vi "Stop Clone VIs (SubVI).vi"(8 "error in":errorcluster, 11 "Data Cluster in":T1={"VI References"=[], "Addresses"=[], "Pilot"=FALSE, "DO Data"=[], "Access Restricted?"=FALSE, "Pilot Control References"=[], "CoPilot Control References"=[], "cRIO Config"=[], "datalog Q"=refnum, "PS_P"={"AI"=[], "DI"=[], "DO"=[], "Serial"=[], "CPU"={"Total Load"=[], "Interrupt Load"=[], "Total Physical"=0.0, "Free Physical"=0.0, "Primary Disk Capacity"=0.0, "Primary Disk Free"=0.0}, "Stop"=FALSE, "DO Channel"=[]}, "PS_S"={"AI"=[], "DI"=[], "DO"=[], "Serial"=[], "CPU"={"Total Load"=[], "Interrupt Load"=[], "Total Physical"=0.0, "Free Physical"=0.0, "Primary Disk Capacity"=0.0, "Primary Disk Free"=0.0}, "Stop"=FALSE, "DO Channel"=[]}, "IDE_P"={"AI"=[], "DI"=[], "DO"=[], "Serial"=[], "CPU"={"Total Load"=[], "Interrupt Load"=[], "Total Physical"=0.0, "Free Physical"=0.0, "Primary Disk Capacity"=0.0, "Primary Disk Free"=0.0}, "Stop"=FALSE, "DO Channel"=[]}, "IDE_S"={"AI"=[], "DI"=[], "DO"=[], "Serial"=[], "CPU"={"Total Load"=[], "Interrupt Load"=[], "Total Physical"=0.0, "Free Physical"=0.0, "Primary Disk Capacity"=0.0, "Primary Disk Free"=0.0}, "Stop"=FALSE, "DO Channel"=[]}, "PDE_P"={"AI"=[], "DI"=[], "DO"=[], "Serial"=[], "CPU"={"Total Load"=[], "Interrupt Load"=[], "Total Physical"=0.0, "Free Physical"=0.0, "Primary Disk Capacity"=0.0, "Primary Disk Free"=0.0}, "Stop"=FALSE, "DO Channel"=[]}, "PDE_S"={"AI"=[], "DI"=[], "DO"=[], "Serial"=[], "CPU"={"Total Load"=[], "Interrupt Load"=[], "Total Physical"=0.0, "Free Physical"=0.0, "Primary Disk Capacity"=0.0, "Primary Disk Free"=0.0}, "Stop"=FALSE, "DO Channel"=[]}, "GUI References"={"Control Names"=[], "Control References"=[]}, "GUI Data"=[], "TCP - Serial"=[], "TCP-Serial Q"=refnum, "TCP Serial Ref"=[], "Data Sets"=[], "Last Data"=[], "Alarm Data"=[], "DI Data"=[], "Ack Data"=[], "Buzzer Data"=[], "Pilot DO"=[], "Co-Pilot DO"=[], "System Down?"=FALSE, "Log Data"=[], "Update Array"=[], "MCC Data Log"=[], "MCC Data Not"=refnum, "Thruster control"=[refnum, refnum, refnum, refnum, refnum, refnum, refnum, refnum, refnum], "waga notifier out"=refnum, "Wago  log"=[], "Thruster Cont"=[0.0, 0.0, 0.0, 0.0, 0.0, 0.0, 0.0, 0.0, 0.0], "Cam Cont"=[FALSE, FALSE, FALSE, FALSE, FALSE, TRUE], "PDE_P TH Cont"={"COM 10"=0.0, "COM 11"=0.0, "COM 12"=0.0, "COM 13"=0.0}, "PDE_S TH Cont"={"COM 10"=0.0, "COM 11"=0.0, "COM 12"=0.0, "COM 13"=0.0}} {"cRIO Config"."AI"."Interface Data"."Timing"."sample mode" items=["Finite Samples"=10178, "Continuous Samples"=10123, "Hardware Timed Single Point"=12522]; "cRIO Config"."Async"."Interface Data"."Data"."Minor Frame Count" min=5 max=8 step=1}) -> (0 "error out":errorcluster)   [LabVIEW 2021]
uses:
  Controls/Host - GUI Data Cluster.ctl
  Analog Output/Controls/AO JSON Data Cluster.ctl
  Analog Output/Controls/AO Interface Data Cluster.ctl
  Analog Output/Controls/AO Channel Configuration Cluster.ctl
  Analog Output/Controls/AO Timing Cluster.ctl
  Digital Output/Controls/DIO Configuration cluster.ctl
  Digital Output/Controls/DIO Interface Data.ctl
  Digital Output/SubVIs/Digital Dynamic Cluster.ctl
  Async JSON Cluster.ctl
  Async Interface Data Cluster.ctl
  Async Serial/Controls/Async Serial Configuration Cluster.ctl
  Async Serial/Controls/Async Frame Info Cluster.ctl
  Async Serial/Controls/Async Message Info Cluster.ctl
  Controls/Host Data Cluster.ctl
  Main Engine/Controls/Main Engine CPU Info.ctl
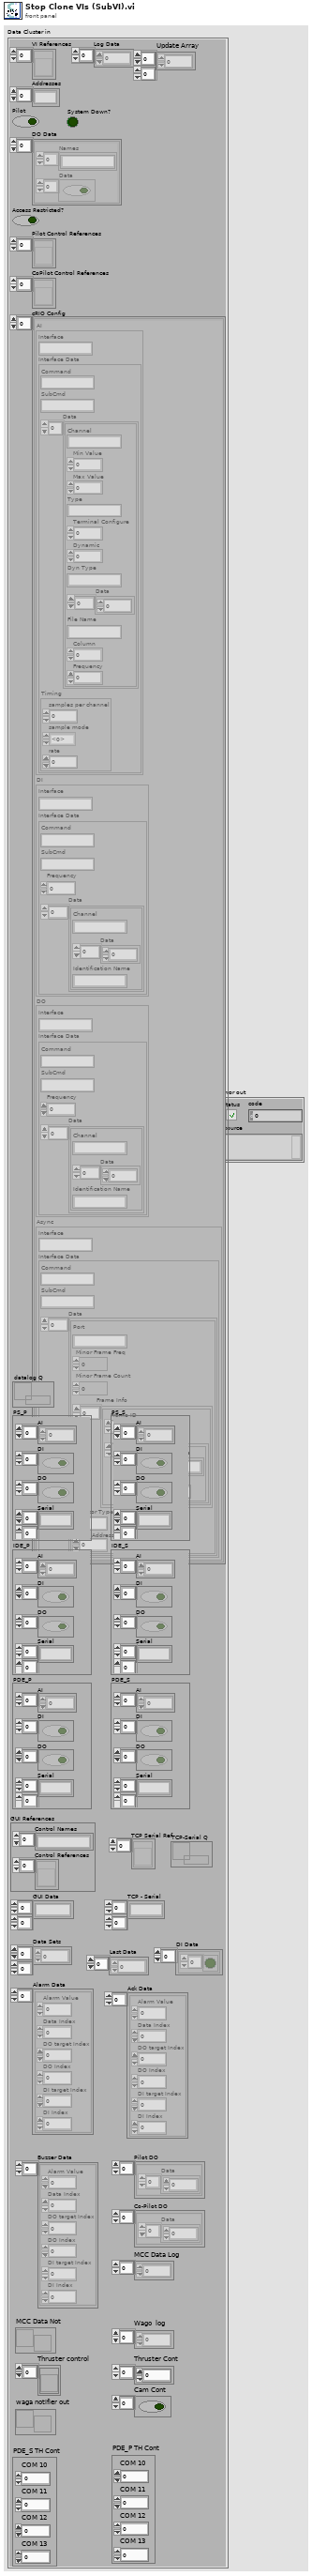
[diagram p1: front panel]
types:
  T1 = typedef "Host - GUI Data Cluster.ctl" = cluster{"VI References":refnum<vi>[], "Addresses":string[], "Pilot":bool, "DO Data":cluster{"Names":string[], "Data":bool[]}[], "Access Restricted?":bool, "Pilot Control References":refnum<vi>[], "CoPilot Control References":refnum<vi>[], "cRIO Config":cluster{"AI":T2, "DI":T6, "DO":T6, "Async":T9}[], "datalog Q":refnum<queue>, "PS_P":T14, "PS_S":T14, "IDE_P":T14, "IDE_S":T14, "PDE_P":T14, "PDE_S":T14, "GUI References":cluster{"Control Names":string[], "Control References":refnum<vi>[]}, "GUI Data":string[][], "TCP - Serial":string[][], "TCP-Serial Q":refnum<queue>, "TCP Serial Ref":refnum<vi>[], "Data Sets":dbl[][], "Last Data":dbl[], "Alarm Data":cluster{"Alarm Value":dbl, "Data Index":i32, "DO target Index":i32, "DO Index":i32, "DI target Index":i32, "DI Index":i32}[], "DI Data":cluster{bool[]}[], "Ack Data":cluster{"Alarm Value":dbl, "Data Index":i32, "DO target Index":i32, "DO Index":i32, "DI target Index":i32, "DI Index":i32}[], "Buzzer Data":cluster{"Alarm Value":dbl, "Data Index":i32, "DO target Index":i32, "DO Index":i32, "DI target Index":i32, "DI Index":i32}[], "Pilot DO":cluster{"Data":i32[]}[], "Co-Pilot DO":cluster{"Data":i32[]}[], "System Down?":bool, "Log Data":dbl[], "Update Array":i32[][], "MCC Data Log":dbl[], "MCC Data Not":refnum<notifier>, "Thruster control":refnum<vi>[], "waga notifier out":refnum<notifier>, "Wago  log":sgl[], "Thruster Cont":dbl[], "Cam Cont":bool[], "PDE_P TH Cont":cluster{"COM 10":dbl, "COM 11":dbl, "COM 12":dbl, "COM 13":dbl}, "PDE_S TH Cont":cluster{"COM 10":dbl, "COM 11":dbl, "COM 12":dbl, "COM 13":dbl}}
  T2 = typedef "AO JSON Data Cluster.ctl" = cluster{"Interface":string, "Interface Data":T3}
  T3 = typedef "AO Interface Data Cluster.ctl" = cluster{"Command":string, "SubCmd":string, "Data":T4[], "Timing":T5}
  T4 = typedef "AO Channel Configuration Cluster.ctl" = cluster{"Channel":string, "Min Value":dbl, "Max Value":dbl, "Type":string, "Terminal Configure":u16, "Dynamic":u8, "Dyn Type":string, "Data":dbl[], "File Name":string, "Column":i32, "Frequency":dbl}
  T5 = typedef "AO Timing Cluster.ctl" = cluster{"samples per channel":i32, "sample mode":i32, "rate":dbl}
  T6 = typedef "DIO Configuration cluster.ctl" = cluster{"Interface":string, "Interface Data":T7}
  T7 = typedef "DIO Interface Data.ctl" = cluster{"Command":string, "SubCmd":string, "Frequency":u16, "Data":T8[]}
  T8 = typedef "Digital Dynamic Cluster.ctl" = cluster{"Channel":string, "Data":u8[], "Identification Name":string}
  T9 = typedef "Async JSON Cluster.ctl" = cluster{"Interface":string, "Interface Data":T10}
  T10 = typedef "Async Interface Data Cluster.ctl" = cluster{"Command":string, "SubCmd":string, "Data":T11[]}
  T11 = typedef "Async Serial Configuration Cluster.ctl" = cluster{"Port":string, "Minor Frame Freq":u16, "Minor Frame Count":u16, "Frame Info":T12[], "Sensor Type":u16, "OIM Address":u16}
  T12 = typedef "Async Frame Info Cluster.ctl" = cluster{"Frame ID":u16, "Message Info":T13[]}
  T13 = typedef "Async Message Info Cluster.ctl" = cluster{"Message":u8[], "Message Name":string}
  T14 = typedef "Host Data Cluster.ctl" = cluster{"AI":dbl[], "DI":bool[], "DO":bool[], "Serial":string[][], "CPU":T15, "Stop":bool, "DO Channel":string[]}
  T15 = typedef "Main Engine CPU Info.ctl" = cluster{"Total Load":u32[], "Interrupt Load":u32[], "Total Physical":dbl, "Free Physical":dbl, "Primary Disk Capacity":dbl, "Primary Disk Free":dbl}
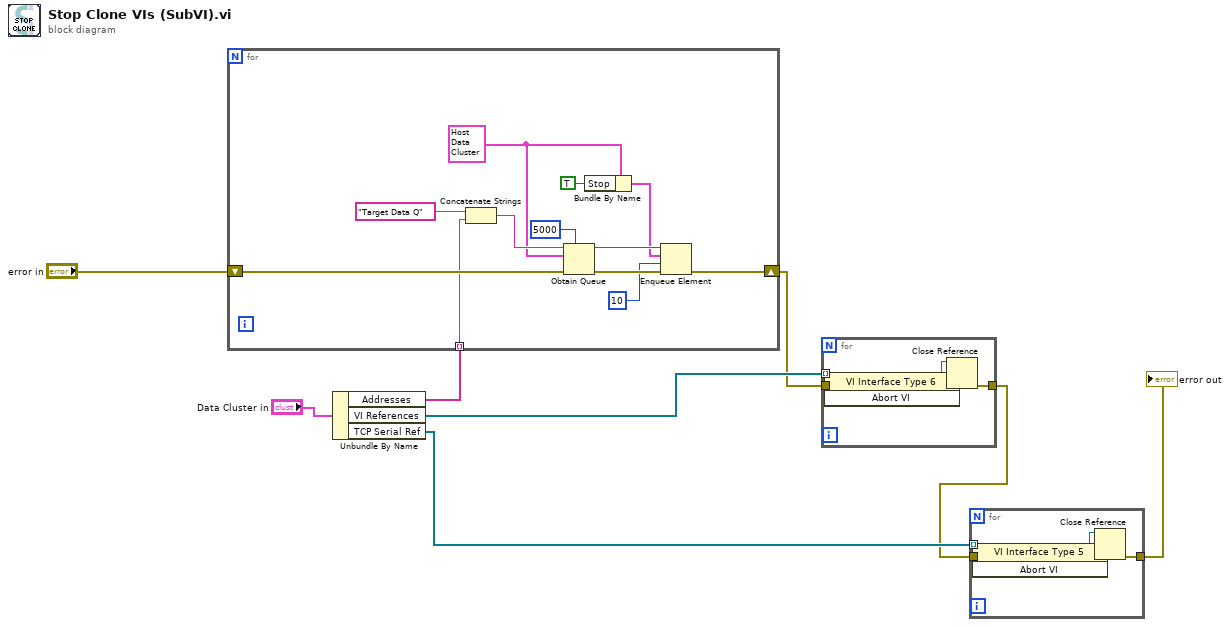
[diagram p0: block diagram]
diagram:
  n1 = Unbundle By Name("Data Cluster in") -> ("Addresses"=w6:string[], "VI References"=w5:refnum<vi>[], "TCP Serial Ref"=w3:refnum<vi>[])
  n2 = for {
    shift-right: [w19] -> w4
    shift-left: "error in" -> [w20]
    tunnel: w6 -> [w10] mode=indexing
    w14 = T14 {"AI"=[-3.29963760152739, -3.28042607250678, -3.30275742266883, -3.28305329003257, -3.29914499819412, -3.27566424083626, -3.29520417157553, -3.26269235518028, -3.14446761533159, -3.13215254239399, -3.16088771377303, -3.13198834142664, -3.16959036650255, -3.151528257494, -3.17188918049567, -3.1431540075152, -3.2208210848143, -3.21425304324317, -3.24479443847459, -3.23132995179905, -3.24922786722435, -3.22706072451644, -3.22311989941762, -3.18896608529332, -3.07895143597999, -3.07616002028715, -3.11064221681751, -3.08551947305428, -3.12459929803547, -3.10916440827463, -3.12197208267327], "DI"=[FALSE, FALSE, FALSE, FALSE, FALSE, FALSE, FALSE, FALSE, FALSE, FALSE, FALSE, FALSE, FALSE, FALSE, FALSE, FALSE, FALSE, FALSE, FALSE, FALSE, FALSE, FALSE, FALSE, FALSE, FALSE, FALSE, FALSE, FALSE, FALSE, FALSE, FALSE, FALSE, FALSE, FALSE, FALSE, FALSE, FALSE, FALSE, FALSE, FALSE, FALSE, FALSE, FALSE, FALSE, FALSE, FALSE, FALSE, FALSE, FALSE, FALSE, FALSE, FALSE, FALSE, FALSE, FALSE, FALSE, FALSE, FALSE, FALSE, FALSE, FALSE, FALSE, FALSE, FALSE], "DO"=[], "Serial"=[], "CPU"={"Total Load"=[], "Interrupt Load"=[], "Total Physical"=0.0, "Free Physical"=0.0, "Primary Disk Capacity"=0.0, "Primary Disk Free"=0.0}, "Stop"=FALSE, "DO Channel"=[]} ("Data Out")
    n3 = Concatenate Strings("Target Data Q" ("name (unnamed)"), w10) -> (w18:string)
    n4 = Obtain Queue(max queue size (-1, unlimited)=5000, name (unnamed)=w18, element data type=w14, error in (no error)=w20) -> (queue out=w15:refnum<queue>, error out=w12:errorcluster)  [unwired: 1 in, 1 out]
    n5 = Bundle By Name(cluster=w14, "Stop"=TRUE) -> (w13:T14)
    n6 = Enqueue Element(queue=w15, element=w13, timeout in ms (-1)=10, error in (no error)=w12) -> (error out=w19:errorcluster)  [unwired: 2 out]
  }
  n7 = for {
    tunnel: w4 -> [w24]
    tunnel: [w22] -> w2
    tunnel: w5 -> [w21] mode=indexing
    n8 = invoke class="VI Interface Type 6" method="Abort VI"(reference=w21, error in=w24) -> (reference out=w25:refnum<vi>, error out=w23:errorcluster)  [unwired: 1 in, 1 out]
    n9 = Close Reference(reference=w25, error in (no error)=w23) -> (error out=w22:errorcluster)
  }
  n10 = for {
    tunnel: w2 -> [w29]
    tunnel: [w27] -> w1
    tunnel: w3 -> [w26] mode=indexing
    n11 = invoke class="VI Interface Type 5" method="Abort VI"(reference=w26, error in=w29) -> (reference out=w30:refnum<vi>, error out=w28:errorcluster)  [unwired: 1 in, 1 out]
    n12 = Close Reference(reference=w30, error in (no error)=w28) -> (error out=w27:errorcluster)
  }
  "error out" <- w1
